vi "asAcq_dataWaitGet_trace.vi"(0 "reference":refnum<class "OSA.lvclass">, 2 "dataType":T1, 5 "error in (no error)":errorcluster, 6 "trace index":u32, 7 "timeout (20000 ms)":i32=20000, 8 "trace set name":string, 9 "error if timeout":bool, 10 "trace set comment":string) -> (13 "timeOut":bool=TRUE, 14 "duplicate reference":refnum<class "OSA.lvclass">, 16 "dataType out":T1, 19 "error out":errorcluster={"status"=TRUE, "code"=1556, "source"="Thorlabs_OSA_64.lvclass:Thorlabs_OSA_64_GetAttributes.vi<ERR>\nThe reference is invalid.\n\n\n<b>Complete call chain:</b>\r\n     Thorlabs_OSA_64.lvclass:Thorlabs_OSA_64_GetAttributes.vi\r\n     Thorlabs_OSA_64.lvclass:asyncAcq_occurenceRef_timeStamp.vi\r\n     Thorlabs_OSA_64.lvclass:asyncAcq_occurenceRef_timeStamp_viServer.vi\r\n     Thorlabs_OSA_64.lvclass:asAcq_dataWait_timeStamp.vi\r\n     Thorlabs_OSA_64.lvclass:asAcq_dataWaitGet.vi"})   [LabVIEW 2010, in "OSA.lvclass"]
doc: "Waits for new data to be available and store retrieved data in a trace buffer, (allocated by FTSLib.dll) - see also data request vis."
uses:
  OSA.lvclass
  typeDef/acq_dataType.ctl
  OSA20X_misc.lvlib
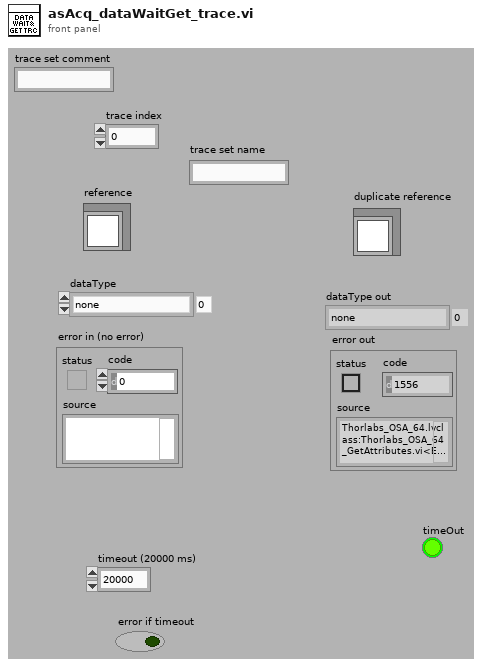
[diagram p1: front panel]
types:
  T1 = typedef "OSA.lvclass/acq_dataType.ctl" = enum16{"none", "interferogram", "spectrum"}
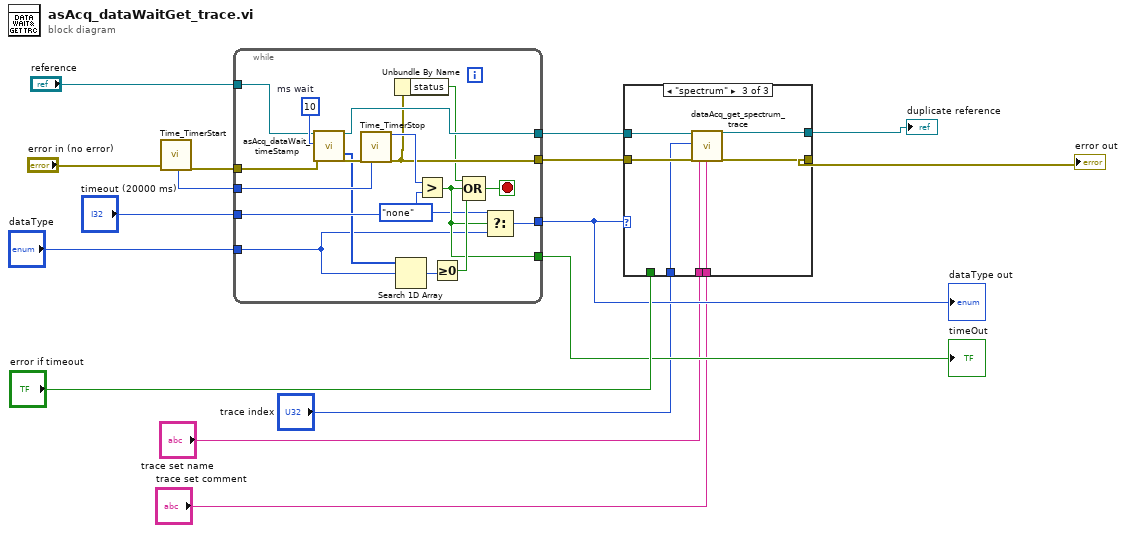
[diagram p0: block diagram]
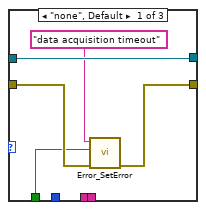
[diagram p2: hidden frame]
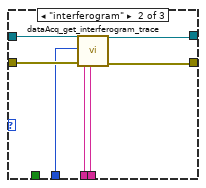
[diagram p3: hidden frame]
diagram:
  n1 = call "Time_TimerStart.vi"("error in (no error)"="error in (no error)") -> ("Start Value (ms timer)"=w13:u32, "error out"=w14:errorcluster)  [unwired: 17 in]
  n2 = while {
    tunnel: [w18] -> w16
    tunnel: [w31] -> w15
    tunnel: w14 -> [w34]
    tunnel: w13 -> [w30]
    tunnel: "timeout (20000 ms)" -> [w28]
    tunnel: "dataType" -> [w19]
    tunnel: "reference" -> [w25]
    tunnel: [w22] -> w4
    tunnel: [w21] -> w5
    stop <- w24 stop-if-true
    w33 = 10  # ms wait
    n3 = call "asAcq_dataWait_timeStamp.vi"("reference"=w25, "ms wait"=w33, "error in (no error)"=w34) -> ("duplicate reference"=w31:refnum<class "OSA.lvclass">, "dataType"=w27:T1[], "error out"=w32:errorcluster)  [unwired: 14 in]
    n4 = call "Time_TimerStop.vi"("error in (no error)"=w32, "Start Value (millisecond timer)"=w30) -> ("Time (millisecond timer)"=w29:i32, "error out"=w18:errorcluster)  [unwired: 16 in]
    n5 = Unbundle By Name(w18) -> ("status"=w17:bool)
    n6 = Search 1D Array(1D array=w27, element=w19) -> (index of element=w26:i32)  [unwired: 1 in]
    n7 = Greater?(x=w29, y=w28) -> (0:w21:bool)
    n8 = Greater Or Equal To 0?(x=w26) -> (x >= 0?=w23:bool)
    n9 = Compound Arithmetic op=OR(w17, w21, w23) -> (w24:bool)
    n10 = Select(t=acq_dataType."none" ("dataType"), s=w21, f=w19) -> (s? t:f=w22:T1)
  }
  "timeOut" <- w5
  "dataType out" <- w4
  n11 = case shown="\"spectrum\"" w4 {
    tunnel: w15 -> [w39 w46 w53]
    tunnel: w16 -> [w37 w44 w52]
    tunnel: [w36 w43 w51] -> w10
    tunnel: [w39 w45 w50] -> w7
    tunnel: "error if timeout" -> [w35 _ _]
    tunnel: "trace set name" -> [_ w42 w49]
    tunnel: "trace index" -> [_ w41 w48]
    tunnel: "trace set comment" -> [_ w40 w47]
    frame "none", Default {
      n12 = call "Error_SetError.vi"("error in"=w37, "status (true)"=w35, "source(\"\")"="data acquisition timeout" ("source(\"\")")) -> ("error out"=w36:errorcluster)  [unwired: 4 in]
    }
    frame "interferogram" {
      n13 = call "dataAcq_get_interferogram_trace.vi"("reference"=w46, "interferogram trace index"=w41, "error in (no error)"=w44, "interferogram trace set name"=w42, "interferogram trace set comment"=w40) -> ("duplicate reference"=w45:refnum<class "OSA.lvclass">, "error out"=w43:errorcluster)  [unwired: 13 in]
    }
    frame "spectrum" {
      n14 = call "dataAcq_get_spectrum_trace.vi"("reference"=w53, "spectrum trace index"=w48, "error in (no error)"=w52, "spectrum trace set name"=w49, "parameter trace set comment"=w47) -> ("duplicate reference"=w50:refnum<class "OSA.lvclass">, "error out"=w51:errorcluster)  [unwired: 13 in]
    }
  }
  "error out" <- w10
  "duplicate reference" <- w7
